vi "ws_templates import template.vi"(8 "error in (no error)":errorcluster, 9 "UploadedFilesList":T1(array[cluster]), 10 "user":string, 11 "Connection Refnum":T4) -> (0 "error out":errorcluster, 1 "template parameters":T2, 2 "New Template Record":T3, 3 "Connection Refnum":T4)   [LabVIEW 2011]
uses:
  SI.LIB/ODBC/SQL Controls/Connection Refnum.ctl
  server/database/Templates/Template Record.ctl
  <vilib>/addons/internet/utils/keyedarr.llb/Keyed Array.ctl
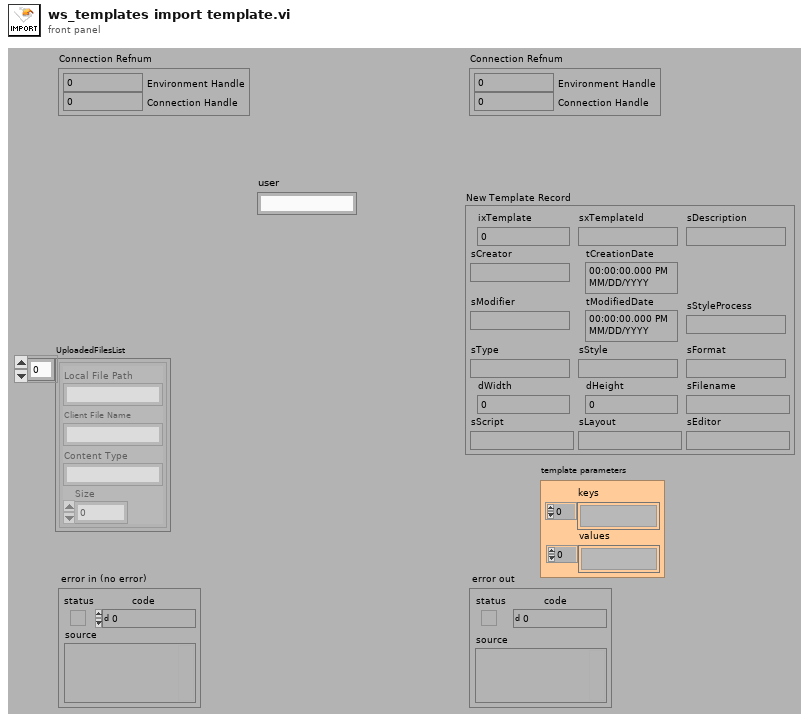
[diagram p1: front panel]
types:
  T1 = cluster{"Local File Path":string, "Client File Name":string, "Content Type":string, "Size":u32}[]
  T2 = typedef "Keyed Array.ctl" = cluster{"keys":string[], "values":string[]}
  T3 = typedef "Template Record.ctl" = cluster{"ixTemplate":i32, "sxTemplateId":string, "sDescription":string, "sCreator":string, "tCreationDate":timestamp, "sModifier":string, "tModifiedDate":timestamp, "sType":string, "sStyle":string, "sFormat":string, "dWidth":dbl, "dHeight":dbl, "sFilename":string, "sScript":string, "sLayout":string, "sEditor":string, "sStyleProcess":string}
  T4 = typedef "Connection Refnum.ctl" = cluster{"Environment Handle":i32, "Connection Handle":i32}
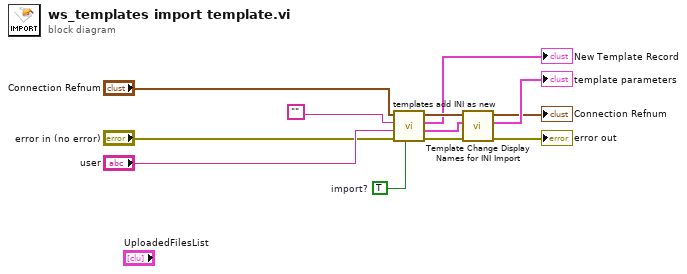
[diagram p0: block diagram]
diagram:
  w7 = TRUE  # import?
  n1 = call "templates add INI as new.vi"("import?"=w7, "error in"="error in (no error)", "user"="user", "INI File Content"="", "Connection Refnum"="Connection Refnum") -> ("error out"=w8:errorcluster, "Parameters"=w10:T2, "updated Template Record"=→"New Template Record":T3, "Connection Refnum 2"=w11:T4)  [unwired: 3 out]
  n2 = call "Template Change Display Names for INI Import.vi"("error in (no error)"=w8, "Parameters"=w10, "Connection Refnum"=w11) -> ("error out"=→"error out":errorcluster, "Parameters 2"=→"template parameters":T2, "Connection Refnum 2"=→"Connection Refnum":T4)  [unwired: 6 out]
